vi "writ2Xml.vi"() -> ()   [LabVIEW 2020, in "simuCalc.lvclass"]
uses:
  simuCalc.lvclass
  <vilib>/Utility/xml.llb/Write to XML File(string).vi
panel:
  in  "Cluster of class private data":T1={"ROI"={"nbrCol"=0, "nbrlign"=0}, "typeSimu"="Random"}
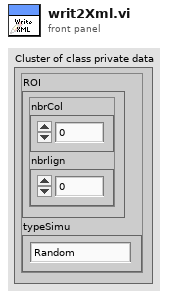
[diagram p1: front panel]
types:
  T1 = cluster{"ROI":cluster{"nbrCol":i32, "nbrlign":i32}, "typeSimu":string}
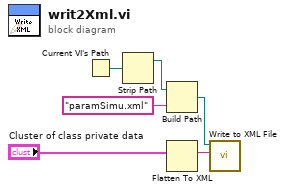
[diagram p0: block diagram]
diagram:
  n1 = Current VI's Path() -> (path=w4:path)
  n2 = Strip Path(path=w4) -> (stripped path=w3:path)  [unwired: 1 out]
  n3 = Build Path(base path=w3, name or relative path="paramSimu.xml") -> (appended path=w5:path)
  n4 = Flatten To XML(6:"Cluster of class private data") -> (2:w1:string)
  n5 = call-poly <vilib>:"Write to XML File.vi"("XML Input"=w1, "XML File Path"=w5) -> ()  [unwired: 7 in, 3 out]
